vi "Run Pre-Render.vi"(8 "Error In":errorcluster, 10 "Abstract Syntax Tree In":refnum<class "Root.lvclass">, 11 "Context In":refnum<class "Compiler.lvclass">) -> (0 "Error Out":errorcluster, 2 "Abstract Syntax Tree Out":refnum<class "Root.lvclass">, 3 "Context Out":refnum<class "Compiler.lvclass">)   [LabVIEW 2018, in "Toolkit.lvlib" / "Compiler.lvclass"]
uses:
  Compiler.lvclass
  Hooks/Render/Process/Process.lvclass
  D:/Users/cfield/Code/Field R&D Services/Labstache/src/Toolkit/Hooks/Hook/Hook.lvclass
  Nodes/Root/Root.lvclass
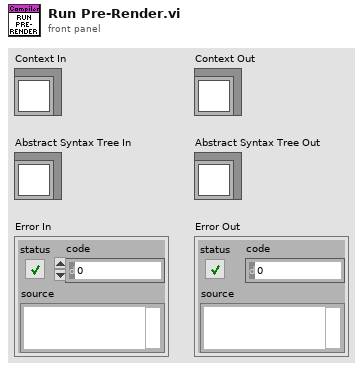
[diagram p1: front panel]
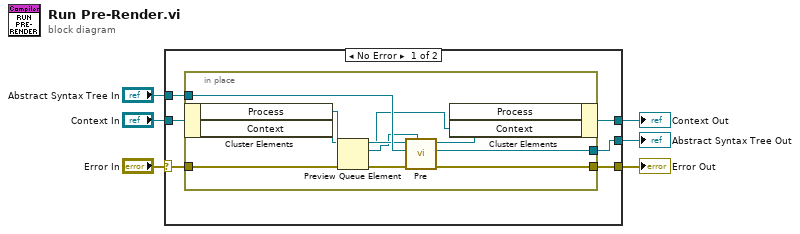
[diagram p0: block diagram]
diagram:
  n1 = case shown="No Error" "Error In" {
    selector: "Error In" -> [w7 w24]
    tunnel: [w12 w25] -> w1
    tunnel: "Context In" -> [w11 w25]
    tunnel: [w10 w23] -> w6
    tunnel: "Abstract Syntax Tree In" -> [w9 w23]
    tunnel: [w8 w24] -> w4
    frame No Error {
      n2 = in-place {
        in-place-border: w7 -> [w22]
        in-place-border: [w21] -> w8
        in-place-border: w9 -> [w20]
        in-place-border: [w19] -> w10
        n3 = in-place-cluster #1(w11) -> ("Process"=w18:refnum<class "Process.lvclass">, "Context"=w15:refnum<queue>)
        n4 = Preview Queue Element(queue=w15, error in (no error)=w22) -> (queue out=w14:refnum<queue>, element=w13:refnum<class "Datum.lvclass">, error out=w16:errorcluster)  [unwired: 1 in, 1 out]
        n5 = call-dynamic "Pre.vi"("Datum"=w13, "Error In"=w16, "Abstract Syntax Tree In"=w20, "Render In"=w18) -> ("Error Out"=w21:errorcluster, "Abstract Syntax Tree Out"=w19:refnum<class "Root.lvclass">, "Render Out"=w17:refnum<class "Process.lvclass">)  [unwired: 5 in]
        n6 = in-place-cluster #1("Process"=w17, "Context"=w14) -> (w12:refnum<class "Compiler.lvclass">)
      }
    }
    frame Error {
    }
  }
  "Abstract Syntax Tree Out" <- w6
  "Error Out" <- w4
  "Context Out" <- w1
